vi "open and format image.vi"(9 "colors":T1={"color diff"=FALSE, "On color"=0, "Off color"=16777215}, 11 "Image path":path) -> (0 "error out":errorcluster, 2 "2D Picture":picture, 3 "1-bit pixmap":bool[][](array[boolean]))   [LabVIEW 2009]
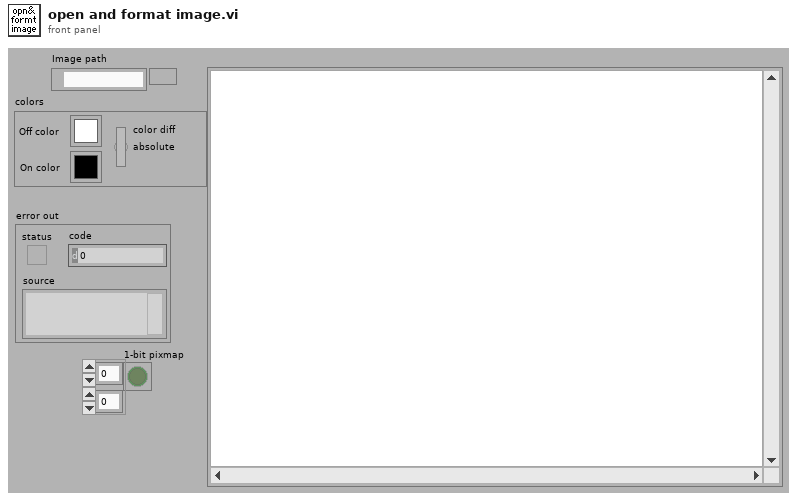
[diagram p1: front panel]
types:
  T1 = cluster{"color diff":bool, "On color":u32, "Off color":u32}
  T2 = typedef "imagedata.ctl" = cluster{"image type":i32, "image depth":i32, "image":u8[], "mask":u8[], "colors":u32[], "Rectangle":cluster{"left":i16, "top":i16, "right":i16, "bottom":i16}}
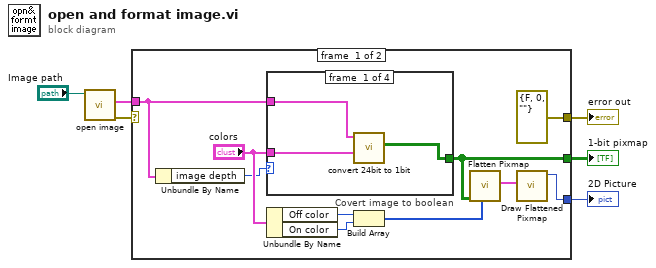
[diagram p0: block diagram]
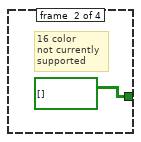
[diagram p2: hidden frame]
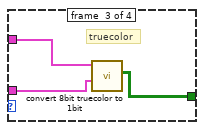
[diagram p3: hidden frame]
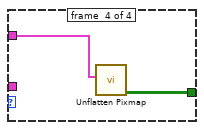
[diagram p4: hidden frame]
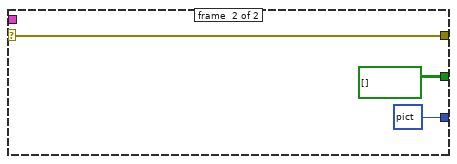
[diagram p5: hidden frame]
diagram:
  n1 = call "open image.vi"("image path"="Image path") -> ("error out"=w2:errorcluster, "image data"=w3:T2)  [unwired: 9 in]
  n2 = case shown="No Error" w2 {
    selector: w2 -> [_ w27]
    tunnel: w3 -> [w16 _]
    tunnel: [w11 picture data[5B] ("new picture")] -> w6
    tunnel: [errorcluster {"status"=FALSE, "code"=0, "source"=""} ("error IO") w27] -> w5
    tunnel: [w8 bool[][] [] ("1-bit pixmap")] -> w1
    frame #0 {
      n3 = Unbundle By Name(w16) -> ("image depth"=w9:i32)
      n4 = case "Covert image to boolean" shown="8" w9 {
        tunnel: [w17 bool[][] [] ("1-bit pixmap") w21 w25] -> w8
        tunnel: w16 -> [w19 _ w23 w24]
        tunnel: "colors" -> [w18 _ w22 _]
        frame #0 {
          n5 = call "convert 24bit to 1bit.vi"("colors"=w18, "image data"=w19) -> ("1-bit pixmap"=w17:bool[][])  [unwired: 8 in, 1 out]
        }
        frame #1 {
          # "16 color\nnot currently\nsupported"
        }
        frame #2 {
          # "truecolor"
          n6 = call "convert 8bit truecolor to 1bit.vi"("colors"=w22, "image data"=w23) -> ("1-bit pixmap"=w21:bool[][])  [unwired: 8 in, 1 out]
        }
        frame #3 {
          n7 = call <vilib>:"Unflatten Pixmap.vi"("image data"=w24) -> ("1-bit pixmap"=w25:bool[][])  [unwired: 4 in, 6 out]
        }
      }
      n8 = Unbundle By Name("colors") -> ("Off color"=w14:u32, "On color"=w13:u32)
      n9 = Build Array(w14, w13) -> (w7:u32[])
      n10 = call <vilib>:"Flatten Pixmap.vi"("colors"=w7, "1-bit pixmap"=w8) -> ("image data"=w12:T2)  [unwired: 9 in]
      n11 = call <vilib>:"Draw Flattened Pixmap.vi"("image data"=w12) -> ("new picture"=w11:picture)  [unwired: 8 in]
    }
    frame #1 {
    }
  }
  "error out" <- w5
  "2D Picture" <- w6
  "1-bit pixmap" <- w1
